vi "SetList_ToString_v4.vi"(3 "Master AO Table":string[][](table), 5 "DDS Table":string[][](table), 6 "Slave  AO Table":string[][](table), 7 "Current Variable settings":T1[](array[typedef]), 8 "SRS Ramps":T4(array[cluster])=[{"lattice ramp"=[{"dt"="", "formula"=""}], "Output"=[{"Time Values"=[0.0, 7.4775e-05, 0.004952823780487805, 0.009830872560975609, 0.014708921341463415, 0.01958697012195122, 0.024465018902439024, 0.02934306768292683, 0.034221116463414636, 0.03909916524390244, 0.04397721402439025, 0.04885526280487805, 0.05373331158536586, 0.05861136036585366, 0.06348940914634146, 0.06836745792682927, 0.07324550670731708, 0.07812355548780488, 0.08300160426829269, 0.0878796530487805, 0.09275770182926829, 0.0976357506097561, 0.10251379939024391, 0.10739184817073172, 0.11226989695121951, 0.11714794573170732, 0.12202599451219513, 0.12690404329268293, 0.13178209207317074, 0.13666014085365855, 0.14153818963414636, 0.14641623841463416, 0.15129428719512195, 0.15617233597560976, 0.16105038475609756, 0.16592843353658537, 0.17080648231707318, 0.175684531097561, 0.1805625798780488, 0.18544062865853658, 0.1903186774390244, 0.1951967262195122, 0.200074775, 0.20014955, 0.20504955, 0.20994955, 0.210024325, 0.710524325, 1.211024325, 1.2110991, 1.2111991, 1.2112991], [-2.42, -2.42, -2.274644675841946, -2.209161629253642, -2.1550360243297555, -2.1059224619056875, -2.059369043262097, -2.0141023350157363, -1.9693429960844966, -1.9245576980378343, -1.8793492014535609, -1.8334007369631589, -1.7864449866349144, -1.7382453890245562, -1.6885840896654052, -1.6372536703029252, -1.5840511006332372, -1.5287730108087192, -1.4712117270212386, -1.4111516989449542, -1.3483660486208333, -1.2826130206804396, -1.2136321308648308, -1.14113980114949, -1.064824236902151, -0.9843392409185628, -0.899296562073762, -0.809256226432418, -0.7137140678937928, -0.6120853153944805, -0.503682519181236, -0.38768515498282585, -0.26309663961745094, -0.1286816451362946, 0.017128703533097003, 0.17638664147159178, 0.35187774884695067, 0.547568099398879, 0.7694813778413232, 1.027657386702481, 1.3414861643128648, 1.7605557393789637, 2.8, 2.8, 2.8, 2.8, 2.8, 2.8, 2.8, -2.42, -2.42, -2.42]}, {"Time Values"=[0.0, 7.4775e-05, 0.004952823780487805, 0.009830872560975609, 0.014708921341463415, 0.01958697012195122, 0.024465018902439024, 0.02934306768292683, 0.034221116463414636, 0.03909916524390244, 0.04397721402439025, 0.04885526280487805, 0.05373331158536586, 0.05861136036585366, 0.06348940914634146, 0.06836745792682927, 0.07324550670731708, 0.07812355548780488, 0.08300160426829269, 0.0878796530487805, 0.09275770182926829, 0.0976357506097561, 0.10251379939024391, 0.10739184817073172, 0.11226989695121951, 0.11714794573170732, 0.12202599451219513, 0.12690404329268293, 0.13178209207317074, 0.13666014085365855, 0.14153818963414636, 0.14641623841463416, 0.15129428719512195, 0.15617233597560976, 0.16105038475609756, 0.16592843353658537, 0.17080648231707318, 0.175684531097561, 0.1805625798780488, 0.18544062865853658, 0.1903186774390244, 0.1951967262195122, 0.200074775, 0.20014955, 0.20504955, 0.20994955, 0.210024325, 0.710524325, 1.211024325, 1.2110991, 1.2111991, 1.2112991], [0.0, -0.0, 0.001911981360536598, 0.004019900016154734, 0.006343835359047381, 0.008905924490689818, 0.011730573093137419, 0.01484468791013227, 0.018277933052562964, 0.022063012569765436, 0.026235981978353178, 0.030836591716105637, 0.03590866579255229, 0.04150051924316252, 0.04766541836368316, 0.05446208810867599, 0.06195527148757928, 0.0702163462869304, 0.07932400499345772, 0.08936500439478239, 0.10043499199819844, 0.11263941713974554, 0.12609453546252153, 0.1409285163325908, 0.15728266374139496, 0.17531276232461152, 0.19519056131922613, 0.21710541059454333, 0.24126606434146913, 0.2679026696014608, 0.2972689585772668, 0.3296446656087423, 0.36533819183711563, 0.40468954294049037, 0.44807356792455355, 0.4959035298202305, 0.5486350423016632, 0.6067704097235386, 0.6708634119196445, 0.7415245793411871, 0.8194270087842359, 0.905312775105144, 1.0, 1.0, 1.0, 1.0, 1.0, 1.0, 1.0, 0.0, 0.0, 0.0]}], "SRS Selection"=enum."Bragg Agilent"}, {"lattice ramp"=[{"dt"="", "formula"=""}], "Output"=[{"Time Values"=[0.0, 7.4775e-05, 0.004952823780487805, 0.009830872560975609, 0.014708921341463415, 0.01958697012195122, 0.024465018902439024, 0.02934306768292683, 0.034221116463414636, 0.03909916524390244, 0.04397721402439025, 0.04885526280487805, 0.05373331158536586, 0.05861136036585366, 0.06348940914634146, 0.06836745792682927, 0.07324550670731708, 0.07812355548780488, 0.08300160426829269, 0.0878796530487805, 0.09275770182926829, 0.0976357506097561, 0.10251379939024391, 0.10739184817073172, 0.11226989695121951, 0.11714794573170732, 0.12202599451219513, 0.12690404329268293, 0.13178209207317074, 0.13666014085365855, 0.14153818963414636, 0.14641623841463416, 0.15129428719512195, 0.15617233597560976, 0.16105038475609756, 0.16592843353658537, 0.17080648231707318, 0.175684531097561, 0.1805625798780488, 0.18544062865853658, 0.1903186774390244, 0.1951967262195122, 0.200074775, 0.20014955, 0.20504955, 0.20994955, 0.210024325, 0.710524325, 1.211024325, 1.2110991, 1.2111991, 1.2112991], [-2.42, -2.42, -2.274644675841946, -2.209161629253642, -2.1550360243297555, -2.1059224619056875, -2.059369043262097, -2.0141023350157363, -1.9693429960844966, -1.9245576980378343, -1.8793492014535609, -1.8334007369631589, -1.7864449866349144, -1.7382453890245562, -1.6885840896654052, -1.6372536703029252, -1.5840511006332372, -1.5287730108087192, -1.4712117270212386, -1.4111516989449542, -1.3483660486208333, -1.2826130206804396, -1.2136321308648308, -1.14113980114949, -1.064824236902151, -0.9843392409185628, -0.899296562073762, -0.809256226432418, -0.7137140678937928, -0.6120853153944805, -0.503682519181236, -0.38768515498282585, -0.26309663961745094, -0.1286816451362946, 0.017128703533097003, 0.17638664147159178, 0.35187774884695067, 0.547568099398879, 0.7694813778413232, 1.027657386702481, 1.3414861643128648, 1.7605557393789637, 2.8, 2.8, 2.8, 2.8, 2.8, 2.8, 2.8, -2.42, -2.42, -2.42]}, {"Time Values"=[0.0, 7.4775e-05, 0.004952823780487805, 0.009830872560975609, 0.014708921341463415, 0.01958697012195122, 0.024465018902439024, 0.02934306768292683, 0.034221116463414636, 0.03909916524390244, 0.04397721402439025, 0.04885526280487805, 0.05373331158536586, 0.05861136036585366, 0.06348940914634146, 0.06836745792682927, 0.07324550670731708, 0.07812355548780488, 0.08300160426829269, 0.0878796530487805, 0.09275770182926829, 0.0976357506097561, 0.10251379939024391, 0.10739184817073172, 0.11226989695121951, 0.11714794573170732, 0.12202599451219513, 0.12690404329268293, 0.13178209207317074, 0.13666014085365855, 0.14153818963414636, 0.14641623841463416, 0.15129428719512195, 0.15617233597560976, 0.16105038475609756, 0.16592843353658537, 0.17080648231707318, 0.175684531097561, 0.1805625798780488, 0.18544062865853658, 0.1903186774390244, 0.1951967262195122, 0.200074775, 0.20014955, 0.20504955, 0.20994955, 0.210024325, 0.710524325, 1.211024325, 1.2110991, 1.2111991, 1.2112991], [0.0, -0.0, 0.001911981360536598, 0.004019900016154734, 0.006343835359047381, 0.008905924490689818, 0.011730573093137419, 0.01484468791013227, 0.018277933052562964, 0.022063012569765436, 0.026235981978353178, 0.030836591716105637, 0.03590866579255229, 0.04150051924316252, 0.04766541836368316, 0.05446208810867599, 0.06195527148757928, 0.0702163462869304, 0.07932400499345772, 0.08936500439478239, 0.10043499199819844, 0.11263941713974554, 0.12609453546252153, 0.1409285163325908, 0.15728266374139496, 0.17531276232461152, 0.19519056131922613, 0.21710541059454333, 0.24126606434146913, 0.2679026696014608, 0.2972689585772668, 0.3296446656087423, 0.36533819183711563, 0.40468954294049037, 0.44807356792455355, 0.4959035298202305, 0.5486350423016632, 0.6067704097235386, 0.6708634119196445, 0.7415245793411871, 0.8194270087842359, 0.905312775105144, 1.0, 1.0, 1.0, 1.0, 1.0, 1.0, 1.0, 0.0, 0.0, 0.0]}], "SRS Selection"=enum."1550 Vertical"}, {"lattice ramp"=[{"dt"="", "formula"=""}], "Output"=[{"Time Values"=[0.0, 7.4775e-05, 0.004952823780487805, 0.009830872560975609, 0.014708921341463415, 0.01958697012195122, 0.024465018902439024, 0.02934306768292683, 0.034221116463414636, 0.03909916524390244, 0.04397721402439025, 0.04885526280487805, 0.05373331158536586, 0.05861136036585366, 0.06348940914634146, 0.06836745792682927, 0.07324550670731708, 0.07812355548780488, 0.08300160426829269, 0.0878796530487805, 0.09275770182926829, 0.0976357506097561, 0.10251379939024391, 0.10739184817073172, 0.11226989695121951, 0.11714794573170732, 0.12202599451219513, 0.12690404329268293, 0.13178209207317074, 0.13666014085365855, 0.14153818963414636, 0.14641623841463416, 0.15129428719512195, 0.15617233597560976, 0.16105038475609756, 0.16592843353658537, 0.17080648231707318, 0.175684531097561, 0.1805625798780488, 0.18544062865853658, 0.1903186774390244, 0.1951967262195122, 0.200074775, 0.20014955, 0.20504955, 0.20994955, 0.210024325, 0.710524325, 1.211024325, 1.2110991, 1.2111991, 1.2112991], [-2.42, -2.42, -2.274644675841946, -2.209161629253642, -2.1550360243297555, -2.1059224619056875, -2.059369043262097, -2.0141023350157363, -1.9693429960844966, -1.9245576980378343, -1.8793492014535609, -1.8334007369631589, -1.7864449866349144, -1.7382453890245562, -1.6885840896654052, -1.6372536703029252, -1.5840511006332372, -1.5287730108087192, -1.4712117270212386, -1.4111516989449542, -1.3483660486208333, -1.2826130206804396, -1.2136321308648308, -1.14113980114949, -1.064824236902151, -0.9843392409185628, -0.899296562073762, -0.809256226432418, -0.7137140678937928, -0.6120853153944805, -0.503682519181236, -0.38768515498282585, -0.26309663961745094, -0.1286816451362946, 0.017128703533097003, 0.17638664147159178, 0.35187774884695067, 0.547568099398879, 0.7694813778413232, 1.027657386702481, 1.3414861643128648, 1.7605557393789637, 2.8, 2.8, 2.8, 2.8, 2.8, 2.8, 2.8, -2.42, -2.42, -2.42]}, {"Time Values"=[0.0, 7.4775e-05, 0.004952823780487805, 0.009830872560975609, 0.014708921341463415, 0.01958697012195122, 0.024465018902439024, 0.02934306768292683, 0.034221116463414636, 0.03909916524390244, 0.04397721402439025, 0.04885526280487805, 0.05373331158536586, 0.05861136036585366, 0.06348940914634146, 0.06836745792682927, 0.07324550670731708, 0.07812355548780488, 0.08300160426829269, 0.0878796530487805, 0.09275770182926829, 0.0976357506097561, 0.10251379939024391, 0.10739184817073172, 0.11226989695121951, 0.11714794573170732, 0.12202599451219513, 0.12690404329268293, 0.13178209207317074, 0.13666014085365855, 0.14153818963414636, 0.14641623841463416, 0.15129428719512195, 0.15617233597560976, 0.16105038475609756, 0.16592843353658537, 0.17080648231707318, 0.175684531097561, 0.1805625798780488, 0.18544062865853658, 0.1903186774390244, 0.1951967262195122, 0.200074775, 0.20014955, 0.20504955, 0.20994955, 0.210024325, 0.710524325, 1.211024325, 1.2110991, 1.2111991, 1.2112991], [0.0, -0.0, 0.001911981360536598, 0.004019900016154734, 0.006343835359047381, 0.008905924490689818, 0.011730573093137419, 0.01484468791013227, 0.018277933052562964, 0.022063012569765436, 0.026235981978353178, 0.030836591716105637, 0.03590866579255229, 0.04150051924316252, 0.04766541836368316, 0.05446208810867599, 0.06195527148757928, 0.0702163462869304, 0.07932400499345772, 0.08936500439478239, 0.10043499199819844, 0.11263941713974554, 0.12609453546252153, 0.1409285163325908, 0.15728266374139496, 0.17531276232461152, 0.19519056131922613, 0.21710541059454333, 0.24126606434146913, 0.2679026696014608, 0.2972689585772668, 0.3296446656087423, 0.36533819183711563, 0.40468954294049037, 0.44807356792455355, 0.4959035298202305, 0.5486350423016632, 0.6067704097235386, 0.6708634119196445, 0.7415245793411871, 0.8194270087842359, 0.905312775105144, 1.0, 1.0, 1.0, 1.0, 1.0, 1.0, 1.0, 0.0, 0.0, 0.0]}], "SRS Selection"=enum."1550 Vertical"}, {"lattice ramp"=[{"dt"="", "formula"=""}], "Output"=[{"Time Values"=[0.0, 7.4775e-05, 0.004952823780487805, 0.009830872560975609, 0.014708921341463415, 0.01958697012195122, 0.024465018902439024, 0.02934306768292683, 0.034221116463414636, 0.03909916524390244, 0.04397721402439025, 0.04885526280487805, 0.05373331158536586, 0.05861136036585366, 0.06348940914634146, 0.06836745792682927, 0.07324550670731708, 0.07812355548780488, 0.08300160426829269, 0.0878796530487805, 0.09275770182926829, 0.0976357506097561, 0.10251379939024391, 0.10739184817073172, 0.11226989695121951, 0.11714794573170732, 0.12202599451219513, 0.12690404329268293, 0.13178209207317074, 0.13666014085365855, 0.14153818963414636, 0.14641623841463416, 0.15129428719512195, 0.15617233597560976, 0.16105038475609756, 0.16592843353658537, 0.17080648231707318, 0.175684531097561, 0.1805625798780488, 0.18544062865853658, 0.1903186774390244, 0.1951967262195122, 0.200074775, 0.20014955, 0.20504955, 0.20994955, 0.210024325, 0.710524325, 1.211024325, 1.2110991, 1.2111991, 1.2112991], [-2.42, -2.42, -2.274644675841946, -2.209161629253642, -2.1550360243297555, -2.1059224619056875, -2.059369043262097, -2.0141023350157363, -1.9693429960844966, -1.9245576980378343, -1.8793492014535609, -1.8334007369631589, -1.7864449866349144, -1.7382453890245562, -1.6885840896654052, -1.6372536703029252, -1.5840511006332372, -1.5287730108087192, -1.4712117270212386, -1.4111516989449542, -1.3483660486208333, -1.2826130206804396, -1.2136321308648308, -1.14113980114949, -1.064824236902151, -0.9843392409185628, -0.899296562073762, -0.809256226432418, -0.7137140678937928, -0.6120853153944805, -0.503682519181236, -0.38768515498282585, -0.26309663961745094, -0.1286816451362946, 0.017128703533097003, 0.17638664147159178, 0.35187774884695067, 0.547568099398879, 0.7694813778413232, 1.027657386702481, 1.3414861643128648, 1.7605557393789637, 2.8, 2.8, 2.8, 2.8, 2.8, 2.8, 2.8, -2.42, -2.42, -2.42]}, {"Time Values"=[0.0, 7.4775e-05, 0.004952823780487805, 0.009830872560975609, 0.014708921341463415, 0.01958697012195122, 0.024465018902439024, 0.02934306768292683, 0.034221116463414636, 0.03909916524390244, 0.04397721402439025, 0.04885526280487805, 0.05373331158536586, 0.05861136036585366, 0.06348940914634146, 0.06836745792682927, 0.07324550670731708, 0.07812355548780488, 0.08300160426829269, 0.0878796530487805, 0.09275770182926829, 0.0976357506097561, 0.10251379939024391, 0.10739184817073172, 0.11226989695121951, 0.11714794573170732, 0.12202599451219513, 0.12690404329268293, 0.13178209207317074, 0.13666014085365855, 0.14153818963414636, 0.14641623841463416, 0.15129428719512195, 0.15617233597560976, 0.16105038475609756, 0.16592843353658537, 0.17080648231707318, 0.175684531097561, 0.1805625798780488, 0.18544062865853658, 0.1903186774390244, 0.1951967262195122, 0.200074775, 0.20014955, 0.20504955, 0.20994955, 0.210024325, 0.710524325, 1.211024325, 1.2110991, 1.2111991, 1.2112991], [0.0, -0.0, 0.001911981360536598, 0.004019900016154734, 0.006343835359047381, 0.008905924490689818, 0.011730573093137419, 0.01484468791013227, 0.018277933052562964, 0.022063012569765436, 0.026235981978353178, 0.030836591716105637, 0.03590866579255229, 0.04150051924316252, 0.04766541836368316, 0.05446208810867599, 0.06195527148757928, 0.0702163462869304, 0.07932400499345772, 0.08936500439478239, 0.10043499199819844, 0.11263941713974554, 0.12609453546252153, 0.1409285163325908, 0.15728266374139496, 0.17531276232461152, 0.19519056131922613, 0.21710541059454333, 0.24126606434146913, 0.2679026696014608, 0.2972689585772668, 0.3296446656087423, 0.36533819183711563, 0.40468954294049037, 0.44807356792455355, 0.4959035298202305, 0.5486350423016632, 0.6067704097235386, 0.6708634119196445, 0.7415245793411871, 0.8194270087842359, 0.905312775105144, 1.0, 1.0, 1.0, 1.0, 1.0, 1.0, 1.0, 0.0, 0.0, 0.0]}], "SRS Selection"=enum."1550 Vertical"}], 9 "Evaporation ramp list":T5[](array[typedef])=[{"Ramp Channels"=[{"Time"="1", "0 Freq. [MHz]"="1", "0 Power [dBm]"="0.1", "1 Freq. [MHz]"="10", "1 Power [dBm]"="0.01"}, {"Time"="2", "0 Freq. [MHz]"="2", "0 Power [dBm]"="0.01", "1 Freq. [MHz]"="12", "1 Power [dBm]"="0.01"}], "2 Freq. [MHz]"="12", "2 Power [dBm]"="1", "3 Freq. [MHz]"="5", "3 Power [dBm]"="1", "Serial Port"="COM1"}], 10 "Slave Staging List":T7[](array[typedef])=[{"Marker"="", "Mode"=enum."Continue", "Output Bits"=[], "Delay (s)"="", "Ramp Step"=1000.0, "String"="", "Line Number"=""}, {"Marker"="", "Mode"=enum."Continue", "Output Bits"=[], "Delay (s)"="", "Ramp Step"=1000.0, "String"="", "Line Number"=""}, {"Marker"="", "Mode"=enum."Continue", "Output Bits"=[], "Delay (s)"="", "Ramp Step"=1000.0, "String"="", "Line Number"=""}, {"Marker"="", "Mode"=enum."Continue", "Output Bits"=[], "Delay (s)"="", "Ramp Step"=1000.0, "String"="", "Line Number"=""}, {"Marker"="", "Mode"=enum."Continue", "Output Bits"=[], "Delay (s)"="", "Ramp Step"=1000.0, "String"="", "Line Number"=""}, {"Marker"="", "Mode"=enum."Continue", "Output Bits"=[], "Delay (s)"="", "Ramp Step"=1000.0, "String"="", "Line Number"=""}, {"Marker"="", "Mode"=enum."Continue", "Output Bits"=[], "Delay (s)"="", "Ramp Step"=1000.0, "String"="", "Line Number"=""}, {"Marker"="", "Mode"=enum."Continue", "Output Bits"=[], "Delay (s)"="", "Ramp Step"=1000.0, "String"="", "Line Number"=""}, {"Marker"="", "Mode"=enum."Continue", "Output Bits"=[], "Delay (s)"="", "Ramp Step"=1000.0, "String"="", "Line Number"=""}, {"Marker"="", "Mode"=enum."Continue", "Output Bits"=[], "Delay (s)"="", "Ramp Step"=1000.0, "String"="", "Line Number"=""}, {"Marker"="", "Mode"=enum."Continue", "Output Bits"=[], "Delay (s)"="", "Ramp Step"=1000.0, "String"="", "Line Number"=""}, {"Marker"="", "Mode"=enum."Continue", "Output Bits"=[], "Delay (s)"="", "Ramp Step"=1000.0, "String"="", "Line Number"=""}, {"Marker"="", "Mode"=enum."Continue", "Output Bits"=[], "Delay (s)"="", "Ramp Step"=1000.0, "String"="", "Line Number"=""}, {"Marker"="", "Mode"=enum."Continue", "Output Bits"=[], "Delay (s)"="", "Ramp Step"=1000.0, "String"="", "Line Number"=""}, {"Marker"="", "Mode"=enum."Continue", "Output Bits"=[], "Delay (s)"="", "Ramp Step"=1000.0, "String"="", "Line Number"=""}, {"Marker"="", "Mode"=enum."Continue", "Output Bits"=[], "Delay (s)"="", "Ramp Step"=1000.0, "String"="", "Line Number"=""}, {"Marker"="", "Mode"=enum."Continue", "Output Bits"=[], "Delay (s)"="", "Ramp Step"=1000.0, "String"="", "Line Number"=""}, {"Marker"="", "Mode"=enum."Continue", "Output Bits"=[], "Delay (s)"="", "Ramp Step"=1000.0, "String"="", "Line Number"=""}, {"Marker"="", "Mode"=enum."Continue", "Output Bits"=[], "Delay (s)"="", "Ramp Step"=1000.0, "String"="", "Line Number"=""}, {"Marker"="", "Mode"=enum."Continue", "Output Bits"=[], "Delay (s)"="", "Ramp Step"=1000.0, "String"="", "Line Number"=""}, {"Marker"="", "Mode"=enum."Continue", "Output Bits"=[], "Delay (s)"="", "Ramp Step"=1000.0, "String"="", "Line Number"=""}, {"Marker"="", "Mode"=enum."Continue", "Output Bits"=[], "Delay (s)"="", "Ramp Step"=1000.0, "String"="", "Line Number"=""}, {"Marker"="", "Mode"=enum."Continue", "Output Bits"=[], "Delay (s)"="", "Ramp Step"=1000.0, "String"="", "Line Number"=""}, {"Marker"="", "Mode"=enum."Continue", "Output Bits"=[], "Delay (s)"="", "Ramp Step"=1000.0, "String"="", "Line Number"=""}, {"Marker"="", "Mode"=enum."Continue", "Output Bits"=[], "Delay (s)"="", "Ramp Step"=1000.0, "String"="", "Line Number"=""}, {"Marker"="", "Mode"=enum."Continue", "Output Bits"=[], "Delay (s)"="", "Ramp Step"=1000.0, "String"="", "Line Number"=""}, {"Marker"="", "Mode"=enum."Continue", "Output Bits"=[], "Delay (s)"="", "Ramp Step"=1000.0, "String"="", "Line Number"=""}, {"Marker"="", "Mode"=enum."Continue", "Output Bits"=[], "Delay (s)"="", "Ramp Step"=1000.0, "String"="", "Line Number"=""}, {"Marker"="", "Mode"=enum."Continue", "Output Bits"=[], "Delay (s)"="", "Ramp Step"=1000.0, "String"="", "Line Number"=""}, {"Marker"="", "Mode"=enum."Continue", "Output Bits"=[], "Delay (s)"="", "Ramp Step"=1000.0, "String"="", "Line Number"=""}, {"Marker"="", "Mode"=enum."Continue", "Output Bits"=[], "Delay (s)"="", "Ramp Step"=1000.0, "String"="", "Line Number"=""}, {"Marker"="", "Mode"=enum."Continue", "Output Bits"=[], "Delay (s)"="", "Ramp Step"=1000.0, "String"="", "Line Number"=""}, {"Marker"="", "Mode"=enum."Continue", "Output Bits"=[], "Delay (s)"="", "Ramp Step"=1000.0, "String"="", "Line Number"=""}, {"Marker"="", "Mode"=enum."Continue", "Output Bits"=[], "Delay (s)"="", "Ramp Step"=1000.0, "String"="", "Line Number"=""}, {"Marker"="", "Mode"=enum."Continue", "Output Bits"=[], "Delay (s)"="", "Ramp Step"=1000.0, "String"="", "Line Number"=""}, {"Marker"="", "Mode"=enum."Continue", "Output Bits"=[], "Delay (s)"="", "Ramp Step"=1000.0, "String"="", "Line Number"=""}, {"Marker"="", "Mode"=enum."Continue", "Output Bits"=[], "Delay (s)"="", "Ramp Step"=1000.0, "String"="", "Line Number"=""}] {"Ramp Step" min=0.0 format="%#_6p"}, 11 "Master Staging List":T7[](array[typedef])=[{"Marker"="", "Mode"=enum."Continue", "Output Bits"=[], "Delay (s)"="", "Ramp Step"=1000.0, "String"="", "Line Number"=""}, {"Marker"="", "Mode"=enum."Continue", "Output Bits"=[], "Delay (s)"="", "Ramp Step"=1000.0, "String"="", "Line Number"=""}, {"Marker"="", "Mode"=enum."Continue", "Output Bits"=[], "Delay (s)"="", "Ramp Step"=1000.0, "String"="", "Line Number"=""}, {"Marker"="", "Mode"=enum."Continue", "Output Bits"=[], "Delay (s)"="", "Ramp Step"=1000.0, "String"="", "Line Number"=""}, {"Marker"="", "Mode"=enum."Continue", "Output Bits"=[], "Delay (s)"="", "Ramp Step"=1000.0, "String"="", "Line Number"=""}, {"Marker"="", "Mode"=enum."Continue", "Output Bits"=[], "Delay (s)"="", "Ramp Step"=1000.0, "String"="", "Line Number"=""}, {"Marker"="", "Mode"=enum."Continue", "Output Bits"=[], "Delay (s)"="", "Ramp Step"=1000.0, "String"="", "Line Number"=""}, {"Marker"="", "Mode"=enum."Continue", "Output Bits"=[], "Delay (s)"="", "Ramp Step"=1000.0, "String"="", "Line Number"=""}, {"Marker"="", "Mode"=enum."Continue", "Output Bits"=[], "Delay (s)"="", "Ramp Step"=1000.0, "String"="", "Line Number"=""}, {"Marker"="", "Mode"=enum."Continue", "Output Bits"=[], "Delay (s)"="", "Ramp Step"=1000.0, "String"="", "Line Number"=""}, {"Marker"="", "Mode"=enum."Continue", "Output Bits"=[], "Delay (s)"="", "Ramp Step"=1000.0, "String"="", "Line Number"=""}, {"Marker"="", "Mode"=enum."Continue", "Output Bits"=[], "Delay (s)"="", "Ramp Step"=1000.0, "String"="", "Line Number"=""}, {"Marker"="", "Mode"=enum."Continue", "Output Bits"=[], "Delay (s)"="", "Ramp Step"=1000.0, "String"="", "Line Number"=""}, {"Marker"="", "Mode"=enum."Continue", "Output Bits"=[], "Delay (s)"="", "Ramp Step"=1000.0, "String"="", "Line Number"=""}, {"Marker"="", "Mode"=enum."Continue", "Output Bits"=[], "Delay (s)"="", "Ramp Step"=1000.0, "String"="", "Line Number"=""}, {"Marker"="", "Mode"=enum."Continue", "Output Bits"=[], "Delay (s)"="", "Ramp Step"=1000.0, "String"="", "Line Number"=""}, {"Marker"="", "Mode"=enum."Continue", "Output Bits"=[], "Delay (s)"="", "Ramp Step"=1000.0, "String"="", "Line Number"=""}, {"Marker"="", "Mode"=enum."Continue", "Output Bits"=[], "Delay (s)"="", "Ramp Step"=1000.0, "String"="", "Line Number"=""}, {"Marker"="", "Mode"=enum."Continue", "Output Bits"=[], "Delay (s)"="", "Ramp Step"=1000.0, "String"="", "Line Number"=""}, {"Marker"="", "Mode"=enum."Continue", "Output Bits"=[], "Delay (s)"="", "Ramp Step"=1000.0, "String"="", "Line Number"=""}, {"Marker"="", "Mode"=enum."Continue", "Output Bits"=[], "Delay (s)"="", "Ramp Step"=1000.0, "String"="", "Line Number"=""}, {"Marker"="", "Mode"=enum."Continue", "Output Bits"=[], "Delay (s)"="", "Ramp Step"=1000.0, "String"="", "Line Number"=""}, {"Marker"="", "Mode"=enum."Continue", "Output Bits"=[], "Delay (s)"="", "Ramp Step"=1000.0, "String"="", "Line Number"=""}, {"Marker"="", "Mode"=enum."Continue", "Output Bits"=[], "Delay (s)"="", "Ramp Step"=1000.0, "String"="", "Line Number"=""}, {"Marker"="", "Mode"=enum."Continue", "Output Bits"=[], "Delay (s)"="", "Ramp Step"=1000.0, "String"="", "Line Number"=""}, {"Marker"="", "Mode"=enum."Continue", "Output Bits"=[], "Delay (s)"="", "Ramp Step"=1000.0, "String"="", "Line Number"=""}, {"Marker"="", "Mode"=enum."Continue", "Output Bits"=[], "Delay (s)"="", "Ramp Step"=1000.0, "String"="", "Line Number"=""}, {"Marker"="", "Mode"=enum."Continue", "Output Bits"=[], "Delay (s)"="", "Ramp Step"=1000.0, "String"="", "Line Number"=""}, {"Marker"="", "Mode"=enum."Continue", "Output Bits"=[], "Delay (s)"="", "Ramp Step"=1000.0, "String"="", "Line Number"=""}, {"Marker"="", "Mode"=enum."Continue", "Output Bits"=[], "Delay (s)"="", "Ramp Step"=1000.0, "String"="", "Line Number"=""}, {"Marker"="", "Mode"=enum."Continue", "Output Bits"=[], "Delay (s)"="", "Ramp Step"=1000.0, "String"="", "Line Number"=""}, {"Marker"="", "Mode"=enum."Continue", "Output Bits"=[], "Delay (s)"="", "Ramp Step"=1000.0, "String"="", "Line Number"=""}, {"Marker"="", "Mode"=enum."Continue", "Output Bits"=[], "Delay (s)"="", "Ramp Step"=1000.0, "String"="", "Line Number"=""}, {"Marker"="", "Mode"=enum."Continue", "Output Bits"=[], "Delay (s)"="", "Ramp Step"=1000.0, "String"="", "Line Number"=""}, {"Marker"="", "Mode"=enum."Continue", "Output Bits"=[], "Delay (s)"="", "Ramp Step"=1000.0, "String"="", "Line Number"=""}, {"Marker"="", "Mode"=enum."Continue", "Output Bits"=[], "Delay (s)"="", "Ramp Step"=1000.0, "String"="", "Line Number"=""}, {"Marker"="", "Mode"=enum."Continue", "Output Bits"=[], "Delay (s)"="", "Ramp Step"=1000.0, "String"="", "Line Number"=""}] {"Ramp Step" min=0.0 format="%#_6p"}) -> (1 "Staging List String":string="# Current Variables\n# \n# Master Staging List\n# Line\tMarker\tOption\tHalt\t0       4       8      12      16      20    AO\tDelay\t\tPoints\t0\t\t1\t\t2\t\t3\t\t4\t\t5\t\t6\t\t7\t\t8\t\t9\t\t10\t\t11\t\t12\t\t13\t\t14\t\t15\t\tComment\n# Slave Staging List\n# Line\tMarker\tOption\tHalt\t0       4       8      12      16      20    AO\tDelay\t\tPoints\t0\t\t1\t\t2\t\t3\t\t4\t\t5\t\t6\t\t7\t\t8\t\t9\t\t10\t\t11\t\t12\t\t13\t\t14\t\t15\t\tComment\n# SRS List\n# \n00\tBragg Agilent\tRamp\teqn\t\tdt\n\t\t\t\t\t\n01\tVertical lattice\tRamp\teqn\t\tdt\n\t\t\t\t\t\n02\tVertical lattice\tRamp\teqn\t\tdt\n\t\t\t\t\t\n03\tVertical lattice\tRamp\teqn\t\tdt\n\t\t\t\t\t\n#\n# Evaporation\n# Port\tFreq2\tPow2\tFreq3\tPow3\nCOM1\t12\t1\t5\t1\t\n\t\t\t1\t1\t0.1\t10\t0.01\n\t\t\t2\t2\t0.01\t12\t0.01\n#Freq0\tPow0\tFreq1\tPow1\nCOM1\t\t\t\t\t\n#Freq0\tPow0\tFreq1\tPow1\nCOM1\t\t\t\t\t\n#Freq0\tPow0\tFreq1\tPow1\nCOM1\t\t\t\t\t\n#Freq0\tPow0\tFreq1\tPow1\nCOM1\t\t\t\t\t\n#Freq0\tPow0\tFreq1\tPow1\nCOM1\t\t\t\t\t\n#Freq0\tPow0\tFreq1\tPow1\nCOM1\t\t\t\t\t\n#Freq0\tPow0\tFreq1\tPow1\nCOM1\t\t\t\t\t\n#Freq0\tPow0\tFreq1\tPow1\nCOM1\t\t\t\t\t\n#Freq0\tPow0\tFreq1\tPow1\nCOM1\t\t\t\t\t\n#Freq0\tPow0\tFreq1\tPow1\nCOM1\t\t\t\t\t\n#Freq0\tPow0\tFreq1\tPow1\n")   [LabVIEW 2012]
uses:
  StagingListEntry.ctt
  StagingListMarkers.ctt
  StagingListOptions.ctt
  EvapRamp.ctt
  EvapRampElement.ctt
  SRSRampControl_v4.ctl
  SRSDevices.ctt
  TypeDefs/Active procedure variables.ctl
  SubVIs.lvlib
  Controls.llb/Controls.lvlib
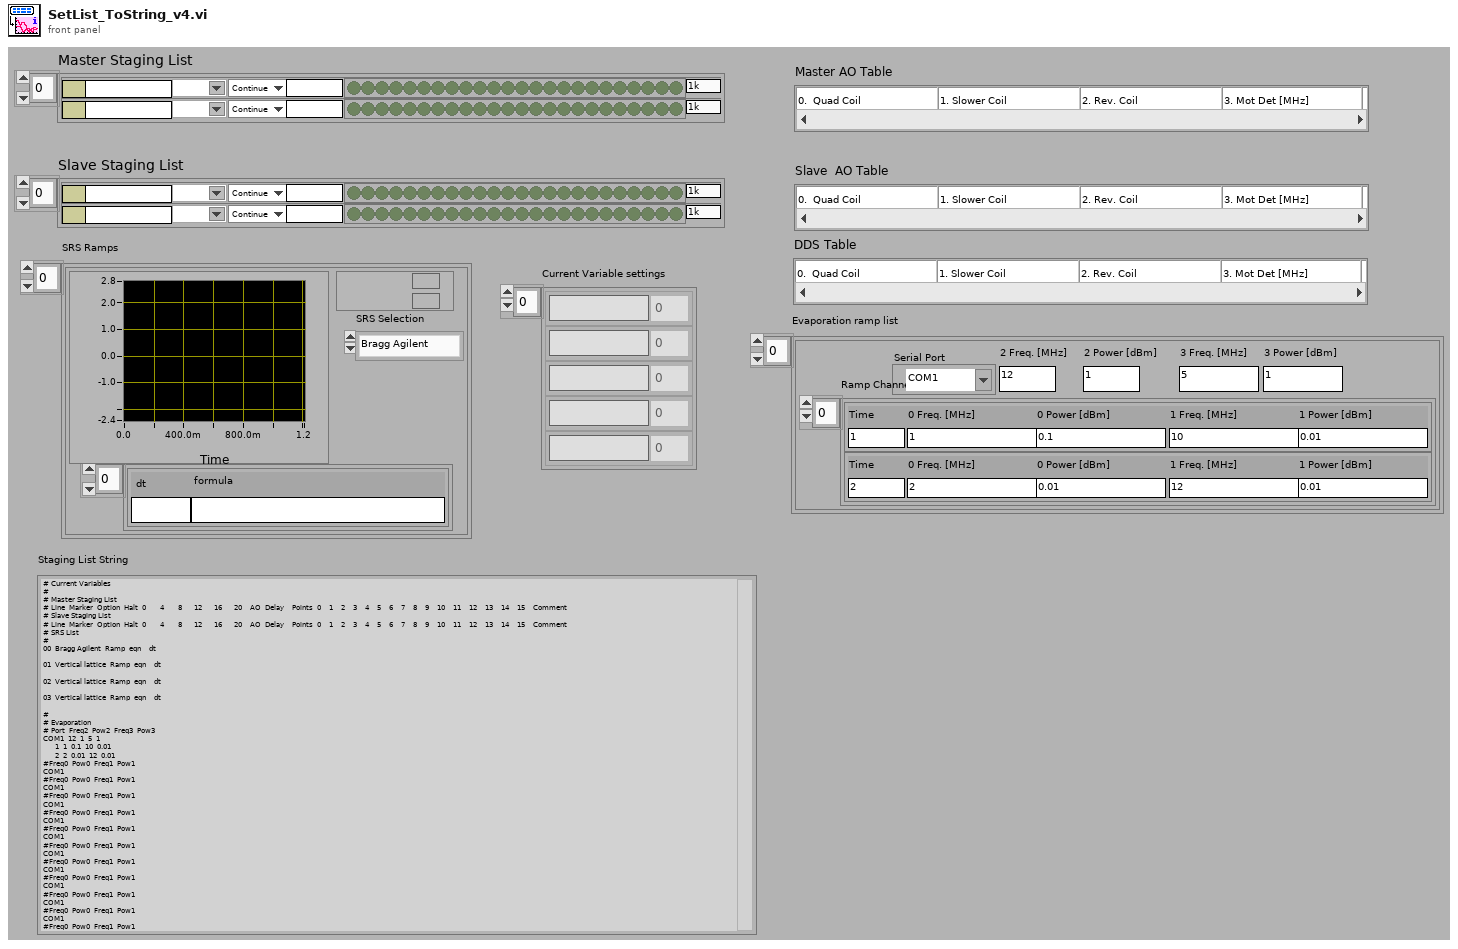
[diagram p1: front panel]
types:
  T1 = typedef "Active procedure variables.ctl" = cluster{"Procedure variable":string, "Value":dbl}
  T2 = typedef "Controls.lvlib/SRSRampControl_v4.ctl" = cluster{"dt":string, "formula":string}
  T3 = typedef "Controls.lvlib/SRSDevices.ctt" = enum16{"1550 Vertical", "Bragg Agilent", "Bragg PTS", "Acc. Intensity"}
  T4 = cluster{"lattice ramp":T2[], "Output":cluster{"Time Values":dbl[], dbl[]}[], "SRS Selection":T3}[]
  T5 = typedef "Controls.lvlib/EvapRamp.ctt" = cluster{"Ramp Channels":T6[], "2 Freq. [MHz]":string, "2 Power [dBm]":string, "3 Freq. [MHz]":string, "3 Power [dBm]":string, "Serial Port":refnum<visa-resource-name>}
  T6 = typedef "Controls.lvlib/EvapRampElement.ctt" = cluster{"Time":string, "0 Freq. [MHz]":string, "0 Power [dBm]":string, "1 Freq. [MHz]":string, "1 Power [dBm]":string}
  T7 = typedef "Controls.lvlib/StagingListEntry.ctt" = cluster{"Marker":T8, "Mode":T9, "Output Bits":bool[], "Delay (s)":string, "Ramp Step":dbl, "String":string, "Line Number":string}
  T8 = typedef "Controls.lvlib/StagingListMarkers.ctt" = string
  T9 = typedef "Controls.lvlib/StagingListOptions.ctt" = enum16{"Continue", "Ramp", "Loop", "EndLoop", "Halt"}
  T10 = cluster{"RF Sweep ?":bool, "RF ramp list":cluster{"Time":dbl, "Frequency [MHz]":dbl, "Power [dBm]":dbl}[]}
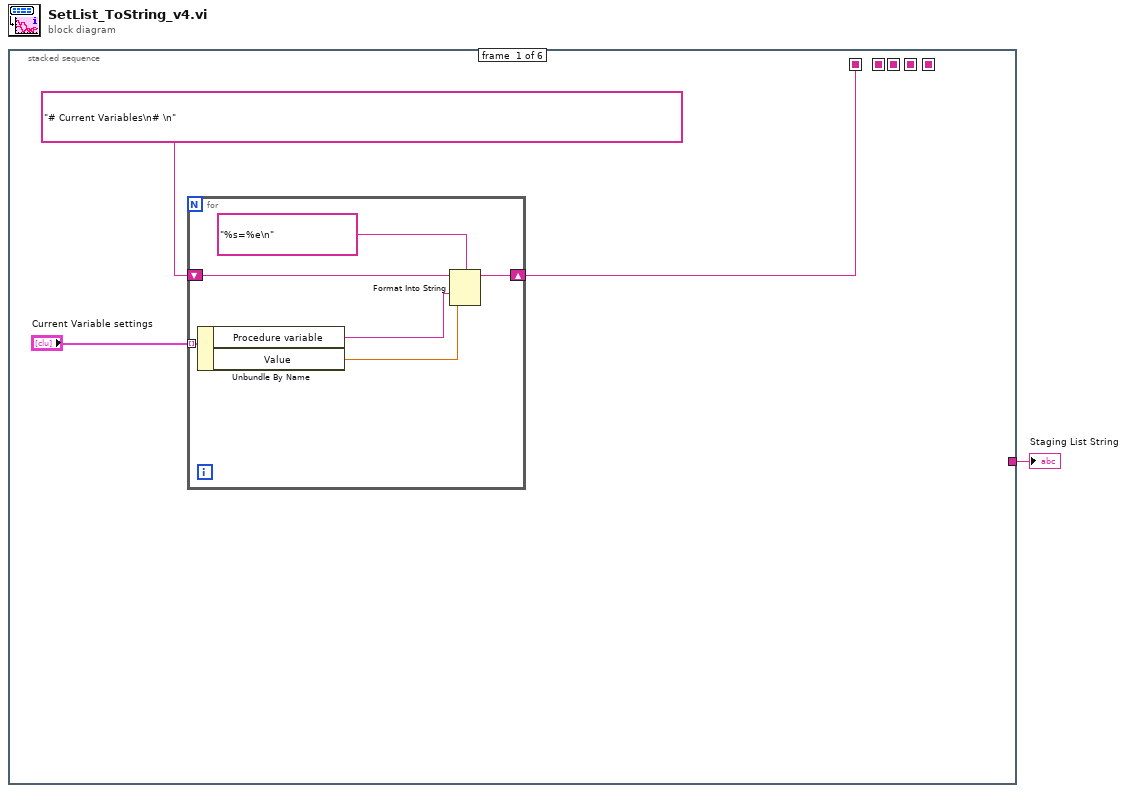
[diagram p0: block diagram]
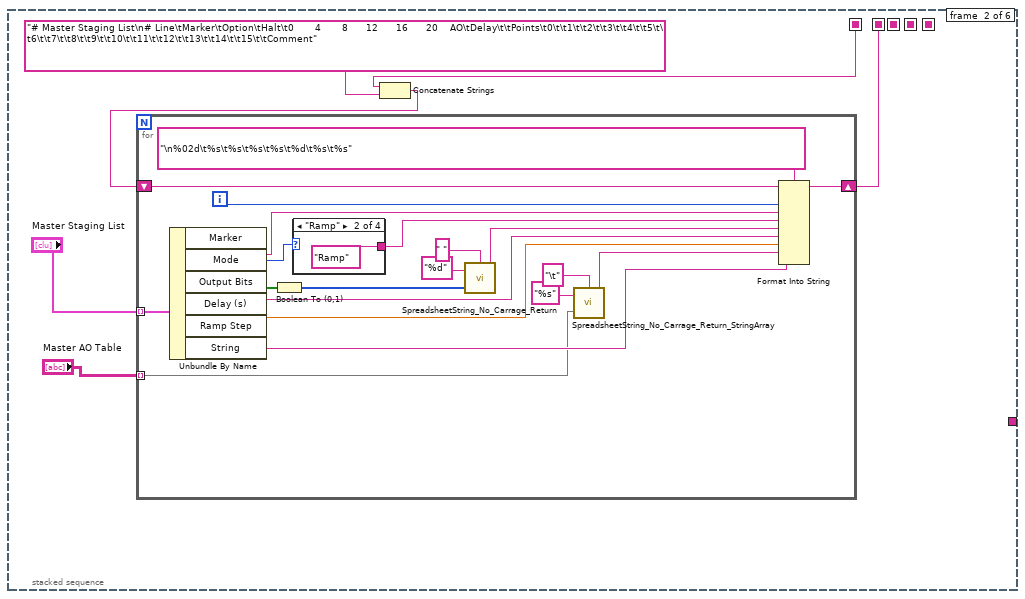
[diagram p2: hidden frame]
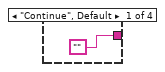
[diagram p3: hidden frame]
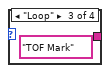
[diagram p4: hidden frame]
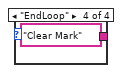
[diagram p5: hidden frame]
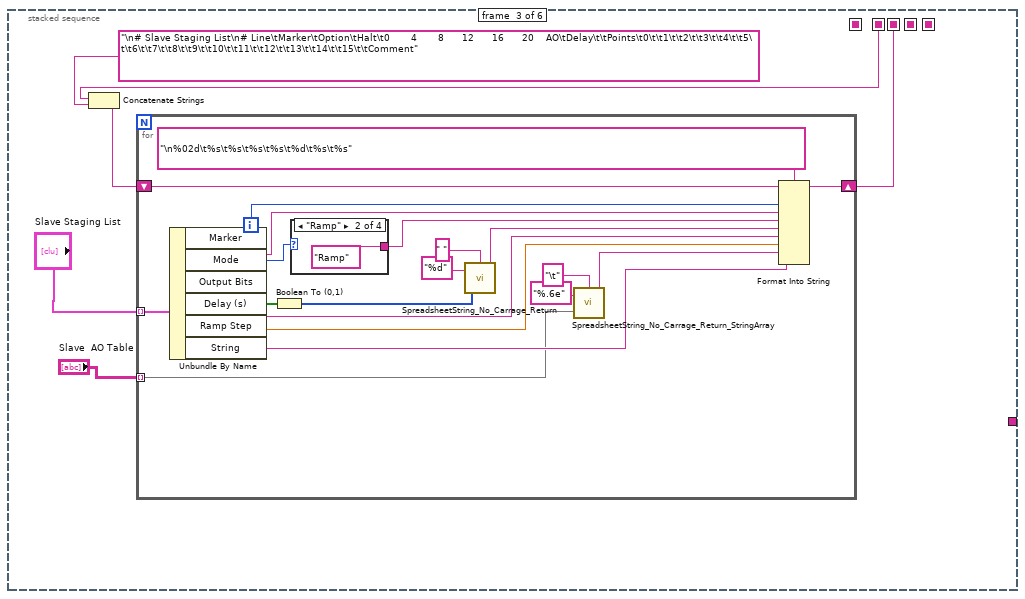
[diagram p6: hidden frame]
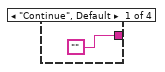
[diagram p7: hidden frame]
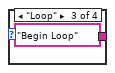
[diagram p8: hidden frame]
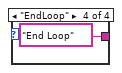
[diagram p9: hidden frame]
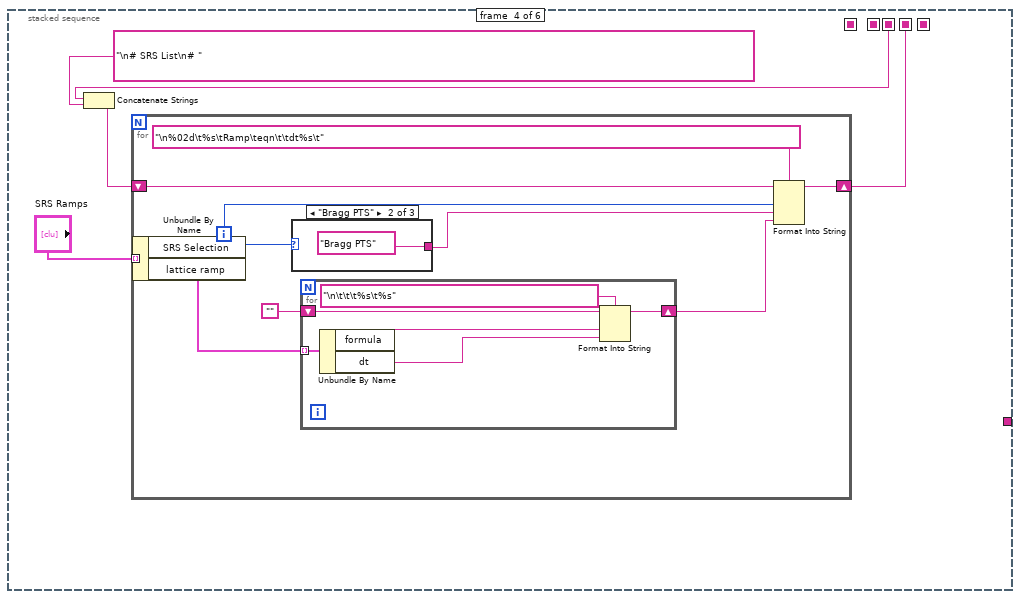
[diagram p10: hidden frame]
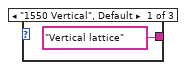
[diagram p11: hidden frame]
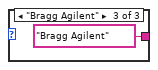
[diagram p12: hidden frame]
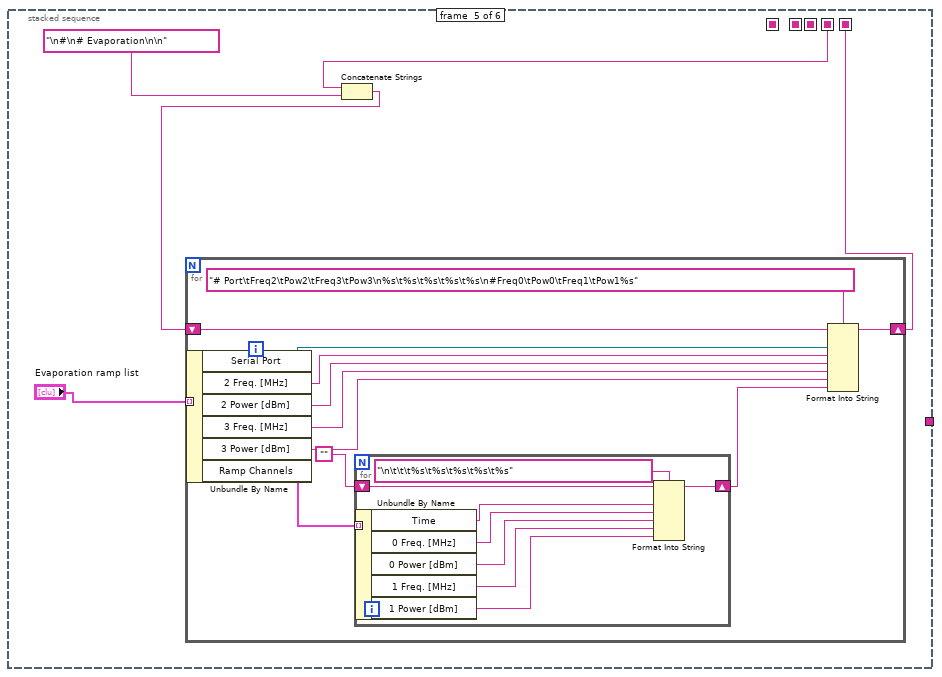
[diagram p13: hidden frame]
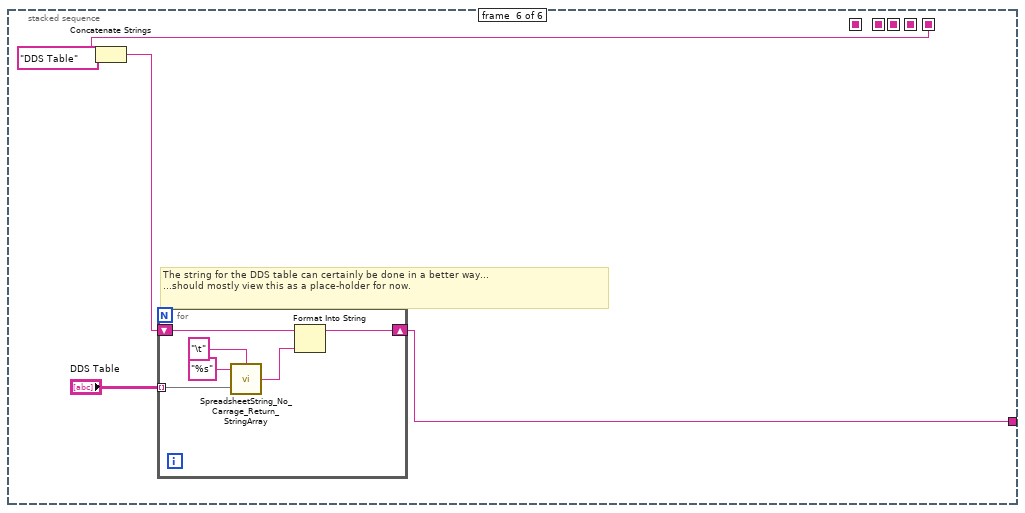
[diagram p14: hidden frame]
diagram:
  n1 = stacked-sequence {
    seq-local: [_ w16 _ _ _ _] -> [_ _ w46 _ _ _]
    seq-local: [_ _ w43 _ _ _] -> [_ _ _ w72 _ _]
    seq-local: [_ _ _ w71 _ _] -> [_ _ _ _ w98 _]
    seq-local: [w2 _ _ _ _ _] -> [_ w12 _ _ _ _]
    seq-local: [_ _ _ _ w95 _] -> [_ _ _ _ _ w125]
    tunnel: [_ _ _ _ _ w121] -> w1
    frame #0 {
      n2 = for {
        tunnel: "Current Variable settings" -> [w7] mode=indexing
        shift-right: [w8] -> w2
        shift-left: "# Current Variables\n# \n" -> [w9]
        n3 = Unbundle By Name(w7) -> ("Procedure variable"=w6:string, "Value"=w5:dbl)
        n4 = Format Into String(format string="%s=%e\n", initial string=w9, w6, w5) -> (resulting string=w8:string)  [unwired: 1 in, 1 out]
      }
    }
    frame #1 {
      (unwired) T10 {"RF Sweep ?"=FALSE, "RF ramp list"=[]} ("Evaporation Params")
      n5 = Concatenate Strings(w12, "# Master Staging List\n# Line\tMarker\tOption\tHalt\t0       4       8      12      16      20    AO\tDelay\t\tPoints\t0\t\t1\t\t2\t\t3\t\t4\t\t5\t\t6\t\t7\t\t8\t\t9\t\t10\t\t11\t\t12\t\t13\t\t14\t\t15\t\tComment") -> (w11:string)
      n6 = for {
        tunnel: "Master Staging List" -> [w36] mode=indexing
        shift-right: [w33] -> w16
        shift-left: w11 -> [w34]
        tunnel: "Master AO Table" -> [w17] mode=indexing
        i -> [w28]
        n7 = Unbundle By Name(w36) -> ("Marker"=w27:T8, "Mode"=w26:T9, "Output Bits"=w29:bool[], "Delay (s)"=w23:string, "Ramp Step"=w22:dbl, "String"=w18:string)
        n8 = Boolean To (0,1)(Boolean=w29) -> (0, 1=w31:i16[])
        n9 = case shown="\"Ramp\"" w26 {
          tunnel: ["" "Ramp" "TOF Mark" "Clear Mark"] -> w25
          frame "Continue", Default {
          }
          frame "Ramp" {
          }
          frame "Loop" {
          }
          frame "EndLoop" {
          }
        }
        n10 = call "SpreadsheetString_No_Carrage_Return.vi"("Deliminator"=" ", "Array"=w31, "Format String"="%d") -> ("spreadsheet string"=w24:string)
        n11 = call "SpreadsheetString_No_Carrage_Return_StringArray.vi"("Deliminator"="\t", "Array"=w17, "Format String"="%s") -> ("spreadsheet string"=w19:string)
        n12 = Format Into String(format string="\n%02d\t%s\t%s\t%s\t%s\t%d\t%s\t%s", initial string=w34, w28, w27, w25, w24, w23, w22, w19, w18) -> (resulting string=w33:string)  [unwired: 1 in, 1 out]
      }
    }
    frame #2 {
      (unwired) T10 {"RF Sweep ?"=FALSE, "RF ramp list"=[]} ("Evaporation Params")
      n13 = Concatenate Strings(w46, "\n# Slave Staging List\n# Line\tMarker\tOption\tHalt\t0       4       8      12      16      20    AO\tDelay\t\tPoints\t0\t\t1\t\t2\t\t3\t\t4\t\t5\t\t6\t\t7\t\t8\t\t9\t\t10\t\t11\t\t12\t\t13\t\t14\t\t15\t\tComment") -> (w44:string)
      n14 = for {
        tunnel: "Slave Staging List" -> [w66] mode=indexing
        shift-right: [w63] -> w43
        shift-left: w44 -> [w64]
        tunnel: "Slave  AO Table" -> [w47] mode=indexing
        i -> [w58]
        n15 = Unbundle By Name(w66) -> ("Marker"=w57:T8, "Mode"=w56:T9, "Output Bits"=w59:bool[], "Delay (s)"=w53:string, "Ramp Step"=w52:dbl, "String"=w48:string)
        n16 = Boolean To (0,1)(Boolean=w59) -> (0, 1=w61:i16[])
        n17 = case shown="\"Ramp\"" w56 {
          tunnel: ["" "Ramp" "Begin Loop" "End Loop"] -> w55
          frame "Continue", Default {
          }
          frame "Ramp" {
          }
          frame "Loop" {
          }
          frame "EndLoop" {
          }
        }
        n18 = call "SpreadsheetString_No_Carrage_Return.vi"("Deliminator"=" ", "Array"=w61, "Format String"="%d") -> ("spreadsheet string"=w54:string)
        n19 = call "SpreadsheetString_No_Carrage_Return_StringArray.vi"("Deliminator"="\t", "Array"=w47, "Format String"="%.6e") -> ("spreadsheet string"=w49:string)
        n20 = Format Into String(format string="\n%02d\t%s\t%s\t%s\t%s\t%d\t%s\t%s", initial string=w64, w58, w57, w55, w54, w53, w52, w49, w48) -> (resulting string=w63:string)  [unwired: 1 in, 1 out]
      }
    }
    frame #3 {
      (unwired) T10 {"RF Sweep ?"=FALSE, "RF ramp list"=[]} ("Evaporation Params")
      n21 = Concatenate Strings(w72, "\n# SRS List\n# ") -> (w74:string)
      n22 = for {
        tunnel: "SRS Ramps" -> [w85] mode=indexing
        shift-right: [w82] -> w71
        shift-left: w74 -> [w83]
        i -> [w81]
        n23 = Unbundle By Name(w85) -> ("SRS Selection"=w79:T3, "lattice ramp"=w77:T2[])
        n24 = case shown="\"Bragg PTS\"" w79 {
          tunnel: ["Vertical lattice" "Bragg PTS" "Bragg Agilent"] -> w80
          frame "1550 Vertical", Default {
          }
          frame "Bragg PTS" {
          }
          frame "Bragg Agilent" {
          }
        }
        n25 = for {
          tunnel: w77 -> [w88] mode=indexing
          shift-right: [w90] -> w76
          shift-left: "" -> [w91]
          n26 = Unbundle By Name(w88) -> ("formula"=w87:string, "dt"=w86:string)
          n27 = Format Into String(format string="\n\t\t\t%s\t%s", initial string=w91, w87, w86) -> (resulting string=w90:string)  [unwired: 1 in, 1 out]
        }
        n28 = Format Into String(format string="\n%02d\t%s\tRamp\teqn\t\tdt%s\t", initial string=w83, w81, w80, w76) -> (resulting string=w82:string)  [unwired: 1 in, 1 out]
      }
    }
    frame #4 {
      n29 = Concatenate Strings(w98, "\n#\n# Evaporation\n\n") -> (w96:string)
      n30 = for {
        tunnel: "Evaporation ramp list" -> [w107] mode=indexing
        shift-right: [w109] -> w95
        shift-left: w96 -> [w110]
        n31 = Unbundle By Name(w107) -> ("Serial Port"=w105:refnum<visa-resource-name>, "2 Freq. [MHz]"=w106:string, "2 Power [dBm]"=w103:string, "3 Freq. [MHz]"=w101:string, "3 Power [dBm]"=w100:string, "Ramp Channels"=w104:T6[])
        n32 = for {
          tunnel: w104 -> [w117] mode=indexing
          shift-right: [w119] -> w102
          shift-left: "" -> [w120]
          n33 = Unbundle By Name(w117) -> ("Time"=w116:string, "0 Freq. [MHz]"=w115:string, "0 Power [dBm]"=w114:string, "1 Freq. [MHz]"=w113:string, "1 Power [dBm]"=w112:string)
          n34 = Format Into String(format string="\n\t\t\t%s\t%s\t%s\t%s\t%s", initial string=w120, w116, w115, w114, w113, w112) -> (resulting string=w119:string)  [unwired: 1 in, 1 out]
        }
        n35 = Format Into String(format string="# Port\tFreq2\tPow2\tFreq3\tPow3\n%s\t%s\t%s\t%s\t%s\n#Freq0\tPow0\tFreq1\tPow1%s", initial string=w110, w105, w106, w103, w101, w100, w102) -> (resulting string=w109:string)  [unwired: 1 in, 1 out]
      }
    }
    frame #5 {
      # "The string for the DDS table can certainly be done in a better way...\n...should mostly view this as a place-holder for now."
      n36 = Concatenate Strings(w125, "DDS Table" ("string")) -> (w122:string)
      n37 = for {
        tunnel: "DDS Table" -> [w129] mode=indexing
        shift-right: [w126] -> w121
        shift-left: w122 -> [w127]
        n38 = call "SpreadsheetString_No_Carrage_Return_StringArray.vi"("Deliminator"="\t", "Array"=w129, "Format String"="%s") -> ("spreadsheet string"=w128:string)
        n39 = Format Into String(initial string=w127, w128) -> (resulting string=w126:string)  [unwired: 2 in, 1 out]
      }
    }
  }
  "Staging List String" <- w1
